vi "Move Older Unmatched Events.vi"(8 "error in (no error)":errorcluster, 11 "Controller in":refnum<class "Controller.lvclass">) -> (0 "error out":errorcluster, 3 "Controller out":refnum<class "Controller.lvclass">)   [LabVIEW 2019, in "Controller.lvlib" / "Controller.lvclass"]
uses:
  Controller.lvclass
  Controller.lvclass/Controller.ctl
  <vilib>/Utility/miscctls.llb/LVMapReplaceAction.ctl
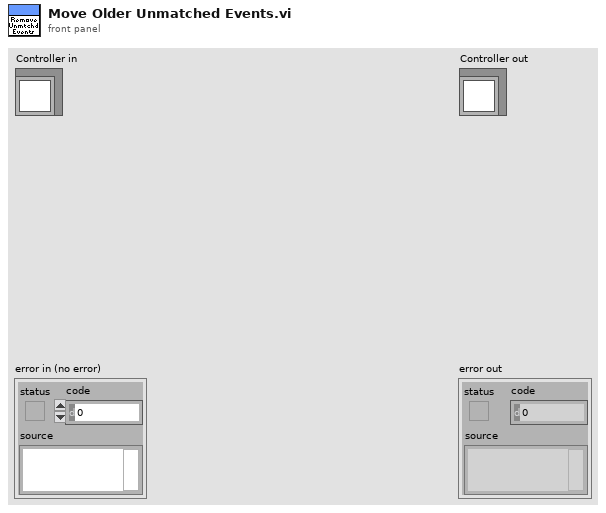
[diagram p1: front panel]
types:
  T1 = typedef "LVMapReplaceAction.ctl" = enum32{"Modify Entry only if found", "Add or Modify Entry", "Delete Entry"}
  T2 = typedef "Muon Detector.lvclass/Event.ctl" = cluster{"Event Count":i32, "Device Timestamp (ms)":i32, "PC Timestamp":timestamp, "ADC Count":i32, "Event Type":u8}
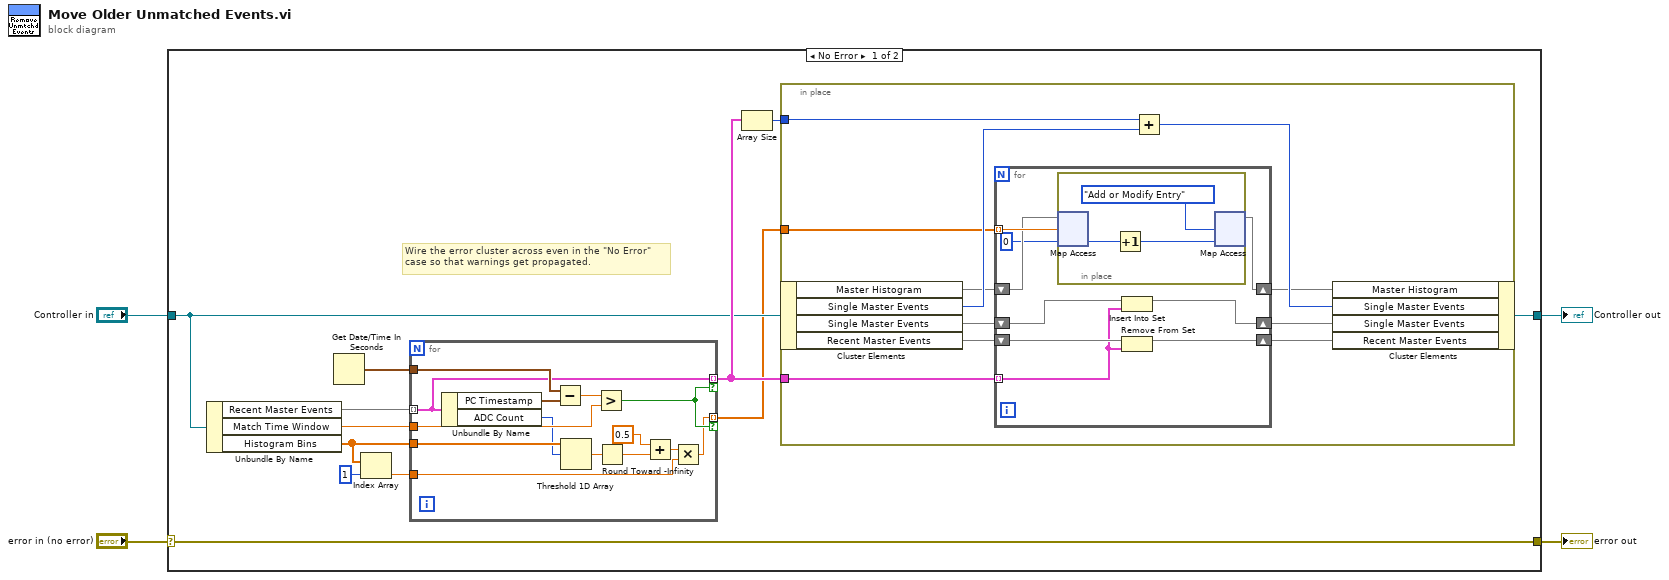
[diagram p0: block diagram]
diagram:
  n1 = case shown="No Error" "error in (no error)" {
    selector: "error in (no error)" -> [w15 w55]
    tunnel: [w15 w55] -> w3
    tunnel: [w14 w54] -> w1
    tunnel: "Controller in" -> [w13 w54]
    frame No Error {
      # "Wire the error cluster across even in the \"No Error\"\ncase so that warnings get propagated."
      n2 = Unbundle By Name(w13) -> ("Recent Master Events"=w12:set{T2}, "Match Time Window"=w10:dbl, "Histogram Bins"=w8:dbl[])
      n3 = Get Date/Time In Seconds() -> (seconds since 1Jan1904=w11:timestamp)
      n4 = Index Array(array=w8, index=1) -> (element=w6:dbl)
      n5 = for {
        tunnel: w12 -> [w26] mode=indexing
        tunnel: w11 -> [w29]
        tunnel: w10 -> [w27]
        tunnel: [w26] -> w16 mode=indexing if=w25
        tunnel: [w18] -> w5 mode=indexing if=w25
        tunnel: w8 -> [w24]
        tunnel: w6 -> [w17]
        n6 = Unbundle By Name(w26) -> ("PC Timestamp"=w30:timestamp, "ADC Count"=w23:i32)
        n7 = Subtract(x=w29, y=w30) -> (x-y=w28:dbl)
        n8 = Threshold 1D Array(2:w23, 3:w24) -> (0:w22:dbl)  [unwired: 1 in]
        n9 = Greater?(x=w28, y=w27) -> (0:w25:bool)
        n10 = Round Toward -Infinity(1:w22) -> (0:w21:dbl)
        n11 = Add(x=0.5, y=w21) -> (x+y=w20:dbl)
        n12 = Multiply(x=w20, y=w17) -> (x*y=w18:dbl)
      }
      n13 = Array Size(array=w16) -> (size(s)=w9:i32)
      n14 = in-place {
        in-place-border: w16 -> [w40]
        in-place-border: w9 -> [w35]
        in-place-border: w5 -> [w31]
        n15 = in-place-cluster #1(w13) -> ("Master Histogram"=w33:map{dbl, i32}, "Single Master Events"=w36:i32, "Single Master Events"=w39:set{T2}, "Recent Master Events"=w41:set{T2})
        n16 = for {
          tunnel: w40 -> [w46] mode=indexing
          shift-right: [w48] -> w38
          shift-left: w41 -> [w49]
          shift-right: [w45] -> w37
          shift-left: w39 -> [w47]
          shift-right: [w43] -> w32
          shift-left: w33 -> [w44]
          tunnel: w31 -> [w50] mode=indexing
          n17 = in-place {
            n18 = in-place-map #2(w44, w50, 0) -> (w52:i32)  [unwired: 1 out]
            n19 = Increment(x=w52) -> (x+1=w51:i32)
            n20 = in-place-map #2(w51, LVMapReplaceAction."Add or Modify Entry" ("action")) -> (w43:map{dbl, i32})  [unwired: 2 out]
          }
          n21 = Insert Into Set(10:w46, 11:w47) -> (3:w45:set{T2})  [unwired: 1 out]
          n22 = Remove From Set(10:w46, 11:w49) -> (3:w48:set{T2})  [unwired: 1 out]
        }
        n23 = Add(x=w35, y=w36) -> (x+y=w34:i32)
        n24 = in-place-cluster #1("Master Histogram"=w32, "Single Master Events"=w34, "Single Master Events"=w37, "Recent Master Events"=w38) -> (w14:refnum<class "Controller.lvclass">)
      }
    }
    frame Error {
    }
  }
  "error out" <- w3
  "Controller out" <- w1
